vi "Draw Boat Icon.vi"(4 "Position":cluster{"X":i32, "Y":i32}, 5 "Boat Bitmap":u32[][](array[numeric]), 6 "Group":string="Boat", 7 "Image In":T1) -> (3 "Image Out":T1)   [LabVIEW 2013]
doc: "Draws the boat icon onto the map at the current location of the boat.\n\n4/5/2014\nMac-I Crowell"
uses:
  <vilib>/vision/Image Controls.llb/IMAQ Image.ctl
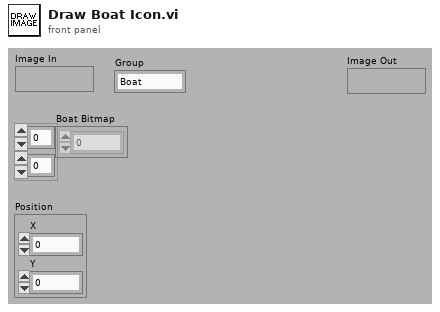
[diagram p1: front panel]
types:
  T1 = typedef "IMAQ Image.ctl" = refnum<image>
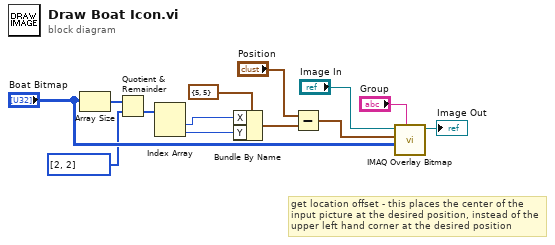
[diagram p0: block diagram]
diagram:
  # "get location offset - this places the center of the input picture at the desired position, instead of the upper left hand corner at the desired position"
  n1 = Array Size(array="Boat Bitmap") -> (size(s)=w7:i32[])
  n2 = Quotient & Remainder(x=w7, y=i32[] [2, 2]) -> (floor(x/y)=w5:i32[])  [unwired: 1 out]
  n3 = Index Array(array=w5) -> (element #1=w2:i32, element #2=w1:i32)  [unwired: 2 in]
  n4 = Bundle By Name(cluster=cluster{"X":i32, "Y":i32} {"X"=5, "Y"=5} ("y"), "X"=w2, "Y"=w1) -> (w4:cluster{"X":i32, "Y":i32})
  n5 = Subtract(x="Position", y=w4) -> (x-y=w13:cluster{"X":i32, "Y":i32})
  n6 = call "IMAQ Overlay Bitmap"("Group"="Group", "Bitmap"="Boat Bitmap", "Top Left Point"=w13, "Image"="Image In") -> ("Image Out"=→"Image Out":T1)  [unwired: 1 in, 6 out]
